vi "3D.vi"() -> ()   [LabVIEW 2018]
uses:
  <vilib>/picture/3D Picture Control/Object/Create Object (name).vi
  <vilib>/picture/3D Picture Control/Object/Add Object (no reference).vi
  <vilib>/picture/3D Picture Control/NI_3D Picture Control.lvlib
panel:
  in  "Station 2 Parameter":cluster{"Length Y":sgl, "Length Z":sgl}={"Length Y"=20.0, "Length Z"=30.0}
  in  "Station 1 Parameter":cluster{"Length X":sgl, "Length Y":sgl}={"Length X"=20.0, "Length Y"=30.0}
  in  "Object Scale":T1={"Length X"=20.0, "Length Y"=30.0, "Length Z"=5.0}
  out "3D 4":refnum<vi>(3d-picture)
  out "3D 3":refnum<vi>(3d-picture)
  out "Camera 2":picture
  out "Camera 1":picture
  out "3D 2":refnum<vi>(3d-picture)
  out "3D 1":refnum<vi>(3d-picture)
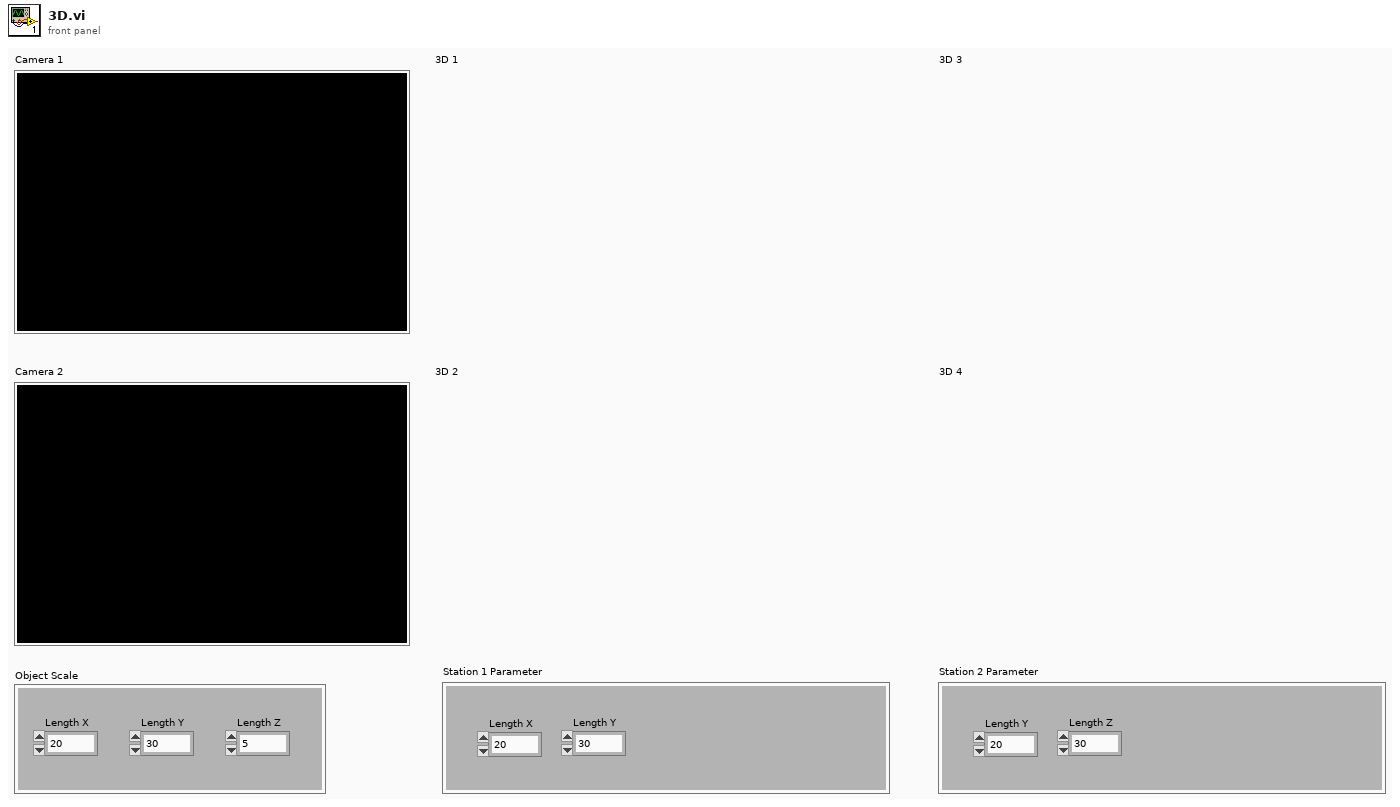
[diagram p1: front panel]
types:
  T1 = cluster{"Length X":sgl, "Length Y":sgl, "Length Z":sgl}
  T2 = enum16{"Inherit Value", "No Culling", "Cull Back Face", "Cull Front Face", "Cull Both Faces"}
  T3 = enum16{"Inherit Value", "Points", "Wireframe", "Polygons"}
  T4 = cluster{"left":i16, "top":i16, "right":i16, "bottom":i16}
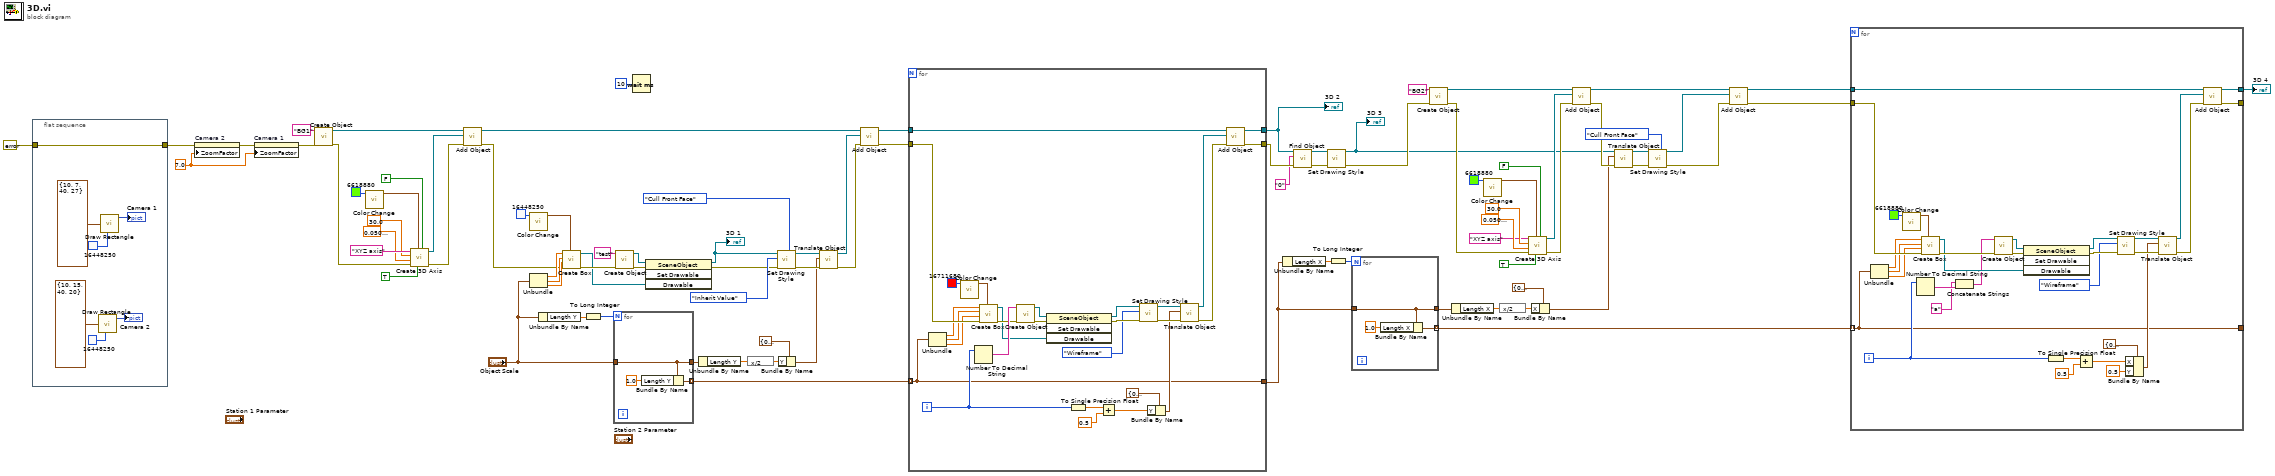
[diagram p0: block diagram]
diagram:
  w43 = sgl 7.0 ("Zoom Factor")
  n1 = flat-sequence {
    tunnel: [w88] -> w41
    tunnel: errorcluster {"status"=FALSE, "code"=0, "source"=""} ("error constant") -> [w88]
    frame #0 {
      n2 = call <vilib>:"Draw Rectangle.vi"("rect"=T4 {"left"=10, "top"=15, "right"=40, "bottom"=20}, "color(black)"=u32 16448250) -> ("new picture"=→"Camera 2":picture)  [unwired: 7 in]
      n3 = call <vilib>:"Draw Rectangle.vi"("rect"=T4 {"left"=10, "top"=7, "right"=40, "bottom"=27}, "color(black)"=u32 16448250) -> ("new picture"=→"Camera 1":picture)  [unwired: 7 in]
    }
  }
  n4 = property on="Camera 2" class="Pict"(error in=w41, "ZoomFactor"=w43) -> (error out=w44:errorcluster)  [unwired: 1 in, 1 out]
  n5 = property on="Camera 1" class="Pict"(error in=w44, "ZoomFactor"=w43) -> (error out=w42:errorcluster)  [unwired: 1 in, 1 out]
  n6 = call-poly <vilib>:"Create Object.vi"("error in (no error)"=w42, "Name"="BG1") -> ("error out"=w63:errorcluster, "Scene:New Object"=w64:refnum<vi>)  [unwired: 8 in]
  n7 = call <vilib>:"Color Change.vi"("Color"=u32 6618880) -> ("RGBA"=w71:cluster{"R":sgl, "G":sgl, "B":sgl, "A":sgl})  [unwired: 10 in]
  n8 = call <vilib>:"Create 3D Axis.vi"("Half plane?"=FALSE, "Axis label?"=TRUE, "Color"=w71, "error in (no error)"=w63, "Radius"=sgl 0.05 ("Character Size"), "Length"=sgl 30.0, "Name"="XYZ axis") -> ("error out"=w62:errorcluster, "New Object Refnum"=w61:refnum<vi>)  [unwired: 3 in]
  n9 = call-poly <vilib>:"Add Object.vi"("error in (no error)"=w62, "New Object In"=w61, "Scene Object In"=w64) -> ("error out"=w60:errorcluster, "Scene Object Out"=w55:refnum<vi>)  [unwired: 7 in]
  n10 = call <vilib>:"Color Change.vi"("Color"=u32 16448250) -> ("RGBA"=w77:cluster{"R":sgl, "G":sgl, "B":sgl, "A":sgl})  [unwired: 10 in]
  n11 = Unbundle("Object Scale") -> ("Length X"=w82:sgl, "Length Y"=w81:sgl, "Length Z"=w80:sgl)
  n12 = Unbundle By Name("Object Scale") -> ("Length Y"=w76:sgl)
  n13 = call <vilib>:"Create Box.vi"("Color"=w77, "error in (no error)"=w60, "Length Z"=w80, "Length Y"=w81, "Length X"=w82) -> ("error out"=w84:errorcluster, "New Box Refnum"=w83:refnum<vi>)  [unwired: 5 in]
  n14 = To Long Integer(number=w76) -> (32bit integer=w75:i32)
  n15 = for {
    N: w75 -> [_]
    tunnel: "Object Scale" -> [w95]
    tunnel: [w96] -> w53 mode=indexing
    tunnel: [w95] -> w52
    n16 = Bundle By Name(cluster=w95, "Length Y"=sgl 1.0) -> (w96:T1)
  }
  n17 = call-poly <vilib>:"Create Object.vi"("error in (no error)"=w84, "Name"="test") -> ("error out"=w86:errorcluster, "Scene:New Object"=w85:refnum<vi>)  [unwired: 8 in]
  n18 = Wait (ms)(milliseconds to wait=u32 10) -> ()  [unwired: 1 out]
  n19 = invoke class="SceneObject" method="Set Drawable"(reference=w85, error in=w86, "Drawable"=w83) -> (reference out=w36:refnum<vi>, error out=w59:errorcluster)  [unwired: 1 in, 2 out]
  "3D 1" <- w36
  n20 = Unbundle By Name(w52) -> ("Length Y"=w51:sgl)
  n21 = expression code="x/2"(w51) -> (w49:sgl)
  n22 = call <vilib>:"Set Drawing Style.vi"("Face Culling Mode"=T2."Cull Front Face", "error in (no error)"=w59, "Mode"=T3."Inherit Value", "Scene Object In"=w36) -> ("error out"=w58:errorcluster, "Scene Object Out"=w57:refnum<vi>)  [unwired: 6 in]
  n23 = Bundle By Name(cluster=cluster{"X":sgl, "Y":sgl, "Z":sgl} {"X"=0.0, "Y"=0.0, "Z"=0.0} ("Translation"), "Y"=w49) -> (w48:cluster{"X":sgl, "Y":sgl, "Z":sgl})
  n24 = call <vilib>:"Translate Object.vi"("error in (no error)"=w58, "Translation"=w48, "Scene.Object In"=w57) -> ("error out"=w56:errorcluster, "Scene.Object Out"=w45:refnum<vi>)  [unwired: 7 in]
  n25 = call-poly <vilib>:"Add Object.vi"("error in (no error)"=w56, "New Object In"=w45, "Scene Object In"=w55) -> ("error out"=w54:errorcluster, "Scene Object Out"=w47:refnum<vi>)  [unwired: 7 in]
  n26 = for {
    tunnel: w53 -> [w98] mode=indexing
    tunnel: w54 -> [w125]
    tunnel: w47 -> [w114]
    tunnel: [w100] -> w37
    tunnel: [w99] -> w39
    tunnel: [w98] -> w33
    i -> [w104]
    n27 = Unbundle(w98) -> ("Length X"=w124:sgl, "Length Y"=w123:sgl, "Length Z"=w122:sgl)
    n28 = call <vilib>:"Color Change.vi"("Color"=u32 16711680) -> ("RGBA"=w120:cluster{"R":sgl, "G":sgl, "B":sgl, "A":sgl})  [unwired: 10 in]
    n29 = Number To Decimal String(number=w104) -> (decimal integer string=w119:string)  [unwired: 1 in]
    n30 = call <vilib>:"Create Box.vi"("Color"=w120, "error in (no error)"=w125, "Length Z"=w122, "Length Y"=w123, "Length X"=w124) -> ("error out"=w118:errorcluster, "New Box Refnum"=w115:refnum<vi>)  [unwired: 5 in]
    n31 = call-poly <vilib>:"Create Object.vi"("error in (no error)"=w118, "Name"=w119) -> ("error out"=w117:errorcluster, "Scene:New Object"=w116:refnum<vi>)  [unwired: 8 in]
    n32 = invoke class="SceneObject" method="Set Drawable"(reference=w116, error in=w117, "Drawable"=w115) -> (reference out=w112:refnum<vi>, error out=w113:errorcluster)  [unwired: 1 in, 2 out]
    n33 = To Single Precision Float(number=w104) -> (single precision float=w103:sgl)
    n34 = Add(x=w103, y=sgl 0.5) -> (x+y=w101:sgl)
    n35 = call <vilib>:"Set Drawing Style.vi"("error in (no error)"=w113, "Mode"=T3."Wireframe", "Scene Object In"=w112) -> ("error out"=w110:errorcluster, "Scene Object Out"=w109:refnum<vi>)  [unwired: 7 in]
    n36 = Bundle By Name(cluster=cluster{"X":sgl, "Y":sgl, "Z":sgl} {"X"=0.0, "Y"=0.0, "Z"=0.0} ("Translation"), "Y"=w101) -> (w107:cluster{"X":sgl, "Y":sgl, "Z":sgl})
    n37 = call <vilib>:"Translate Object.vi"("error in (no error)"=w110, "Translation"=w107, "Scene.Object In"=w109) -> ("error out"=w106:errorcluster, "Scene.Object Out"=w105:refnum<vi>)  [unwired: 7 in]
    n38 = call-poly <vilib>:"Add Object.vi"("error in (no error)"=w106, "New Object In"=w105, "Scene Object In"=w114) -> ("error out"=w99:errorcluster, "Scene Object Out"=w100:refnum<vi>)  [unwired: 7 in]
  }
  "3D 2" <- w37
  n39 = Unbundle By Name(w33) -> ("Length X"=w32:sgl)
  n40 = call <vilib>:"Find Object.vi"("error in (no error)"=w39, "Object Name"="0", "Scene Refnum"=w37) -> ("error out"=w35:errorcluster, "Object Refnum"=w34:refnum<vi>)  [unwired: 7 in]
  n41 = call <vilib>:"Set Drawing Style.vi"("error in (no error)"=w35, "Scene Object In"=w34) -> ("error out"=w15:errorcluster, "Scene Object Out"=w12:refnum<vi>)  [unwired: 8 in]
  "3D 3" <- w12
  n42 = To Long Integer(number=w32) -> (32bit integer=w31:i32)
  n43 = for {
    N: w31 -> [_]
    tunnel: w33 -> [w126]
    tunnel: [w127] -> w6 mode=indexing
    tunnel: [w126] -> w28
    n44 = Bundle By Name(cluster=w126, "Length X"=sgl 1.0 ("Length Y")) -> (w127:T1)
  }
  n45 = call-poly <vilib>:"Create Object.vi"("error in (no error)"=w15, "Name"="BG2") -> ("error out"=w14:errorcluster, "Scene:New Object"=w13:refnum<vi>)  [unwired: 8 in]
  n46 = Unbundle By Name(w28) -> ("Length X"=w29:sgl)
  n47 = call <vilib>:"Color Change.vi"("Color"=u32 6618880) -> ("RGBA"=w22:cluster{"R":sgl, "G":sgl, "B":sgl, "A":sgl})  [unwired: 10 in]
  n48 = expression code="x/2"(w29) -> (w30:sgl)
  n49 = call <vilib>:"Create 3D Axis.vi"("Half plane?"=FALSE, "Axis label?"=TRUE, "Color"=w22, "error in (no error)"=w14, "Radius"=sgl 0.05 ("Character Size"), "Length"=sgl 30.0, "Name"="XYZ axis") -> ("error out"=w18:errorcluster, "New Object Refnum"=w19:refnum<vi>)  [unwired: 3 in]
  n50 = Bundle By Name(cluster=cluster{"X":sgl, "Y":sgl, "Z":sgl} {"X"=0.0, "Y"=0.0, "Z"=0.0} ("Translation"), "X"=w30) -> (w8:cluster{"X":sgl, "Y":sgl, "Z":sgl})
  n51 = call-poly <vilib>:"Add Object.vi"("error in (no error)"=w18, "New Object In"=w19, "Scene Object In"=w13) -> ("error out"=w17:errorcluster, "Scene Object Out"=w11:refnum<vi>)  [unwired: 7 in]
  n52 = call <vilib>:"Translate Object.vi"("error in (no error)"=w17, "Translation"=w8, "Scene.Object In"=w12) -> ("error out"=w5:errorcluster, "Scene.Object Out"=w4:refnum<vi>)  [unwired: 7 in]
  n53 = call <vilib>:"Set Drawing Style.vi"("Face Culling Mode"=T2."Cull Front Face", "error in (no error)"=w5, "Scene Object In"=w4) -> ("error out"=w3:errorcluster, "Scene Object Out"=w2:refnum<vi>)  [unwired: 7 in]
  n54 = call-poly <vilib>:"Add Object.vi"("error in (no error)"=w3, "New Object In"=w2, "Scene Object In"=w11) -> ("error out"=w9:errorcluster, "Scene Object Out"=w10:refnum<vi>)  [unwired: 7 in]
  n55 = for {
    tunnel: w6 -> [w133] mode=indexing
    tunnel: w9 -> [w159]
    tunnel: w10 -> [w149]
    tunnel: [w135] -> w7
    tunnel: [w134] -> _
    tunnel: [w133] -> _
    i -> [w139]
    n56 = Unbundle(w133) -> ("Length X"=w158:sgl, "Length Y"=w157:sgl, "Length Z"=w156:sgl)
    n57 = call <vilib>:"Color Change.vi"("Color"=u32 6618880) -> ("RGBA"=w154:cluster{"R":sgl, "G":sgl, "B":sgl, "A":sgl})  [unwired: 10 in]
    n58 = Number To Decimal String(number=w139) -> (decimal integer string=w132:string)  [unwired: 1 in]
    n59 = call <vilib>:"Create Box.vi"("Color"=w154, "error in (no error)"=w159, "Length Z"=w156, "Length Y"=w157, "Length X"=w158) -> ("error out"=w153:errorcluster, "New Box Refnum"=w150:refnum<vi>)  [unwired: 5 in]
    n60 = Concatenate Strings("a" ("string"), w132) -> (w130:string)
    n61 = call-poly <vilib>:"Create Object.vi"("error in (no error)"=w153, "Name"=w130) -> ("error out"=w152:errorcluster, "Scene:New Object"=w151:refnum<vi>)  [unwired: 8 in]
    n62 = invoke class="SceneObject" method="Set Drawable"(reference=w151, error in=w152, "Drawable"=w150) -> (reference out=w147:refnum<vi>, error out=w148:errorcluster)  [unwired: 1 in, 2 out]
    n63 = To Single Precision Float(number=w139) -> (single precision float=w138:sgl)
    n64 = Add(x=w138, y=sgl 0.5) -> (x+y=w136:sgl)
    n65 = call <vilib>:"Set Drawing Style.vi"("error in (no error)"=w148, "Mode"=T3."Wireframe", "Scene Object In"=w147) -> ("error out"=w145:errorcluster, "Scene Object Out"=w144:refnum<vi>)  [unwired: 7 in]
    n66 = Bundle By Name(cluster=cluster{"X":sgl, "Y":sgl, "Z":sgl} {"X"=0.0, "Y"=0.0, "Z"=0.0} ("Translation"), "X"=w136, "Y"=sgl 0.5) -> (w142:cluster{"X":sgl, "Y":sgl, "Z":sgl})
    n67 = call <vilib>:"Translate Object.vi"("error in (no error)"=w145, "Translation"=w142, "Scene.Object In"=w144) -> ("error out"=w141:errorcluster, "Scene.Object Out"=w140:refnum<vi>)  [unwired: 7 in]
    n68 = call-poly <vilib>:"Add Object.vi"("error in (no error)"=w141, "New Object In"=w140, "Scene Object In"=w149) -> ("error out"=w134:errorcluster, "Scene Object Out"=w135:refnum<vi>)  [unwired: 7 in]
  }
  "3D 4" <- w7
